vi "Log.vi"(10 "Log Packet":T1, 11 "String Log Sink in":refnum<class "String Log Sink.lvclass">) -> (0 "error out":errorcluster, 3 "String Log Sink out":refnum<class "String Log Sink.lvclass">)   [LabVIEW 2019, in "String Log Sink.lvclass"]
uses:
  <vilib>/gpm_packages/@cs/event-logger/Source/String Log Sink/String Log Sink.lvclass
  <vilib>/gpm_packages/@cs/event-logger/Source/Composed Log/Types/Log Packet.ctl
  <vilib>/gpm_packages/@cs/event-logger/Source/Composed Log/Types/Log Level.ctl
  <vilib>/gpm_packages/@cs/event-logger/Source/String Log Sink/String Log Sink.lvclass/String Log Sink.ctl
  <vilib>/gpm_packages/@cs/event-logger/Source/IStringFormat/IStringFormat.lvclass
  <vilib>/gpm_packages/@cs/event-logger/Source/Composed Log/Composed Log.lvlib
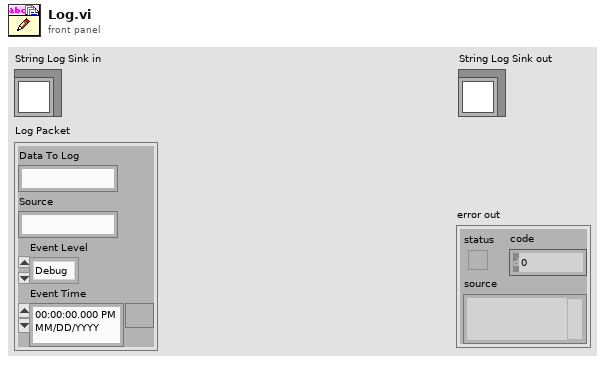
[diagram p1: front panel]
types:
  T1 = typedef "Composed Log.lvlib/Log Packet.ctl" = cluster{"Data To Log":string, "Source":string, "Event Level":T2, "Event Time":timestamp}
  T2 = typedef "Composed Log.lvlib/Log Level.ctl" = enum16{"Debug", "Info", "Warning", "Error", "Critical"}
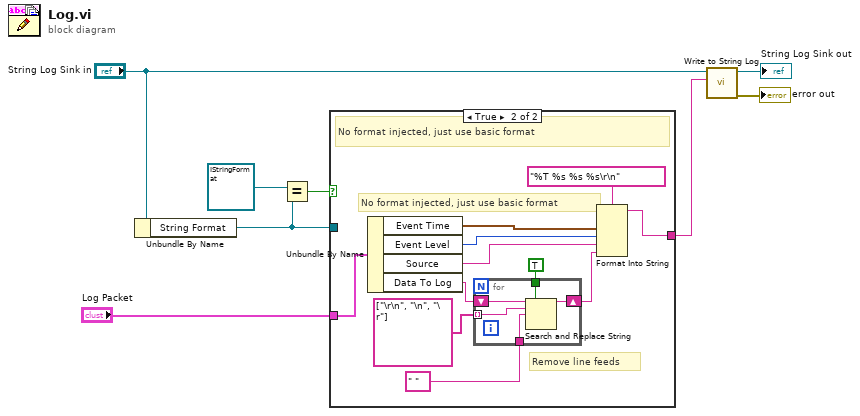
[diagram p0: block diagram]
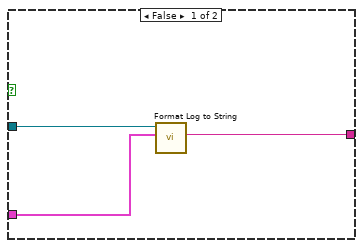
[diagram p2: hidden frame]
diagram:
  n1 = Unbundle By Name("String Log Sink in") -> ("String Format"=w6:refnum<class "IStringFormat.lvclass">)
  n2 = Equal?(x=refnum<class "IStringFormat.lvclass"> refnum ("y"), y=w6) -> (x = y?=w7:bool)
  n3 = case shown="True" w7 {
    tunnel: w6 -> [w11 _]
    tunnel: "Log Packet" -> [w10 w13]
    tunnel: [w9 w12] -> w2
    frame False {
      n4 = call-dynamic "Format Log to String.vi"("Log Packet"=w10, "IStringFormat in"=w11) -> ("Log Entry"=w9:string)  [unwired: 8 in, 1 out]
    }
    frame True {
      # "Remove line feeds"
      # "No format injected, just use basic format"
      # "No format injected, just use basic format"
      n5 = Unbundle By Name(w13) -> ("Event Time"=w22:timestamp, "Event Level"=w20:T2, "Source"=w19:string, "Data To Log"=w18:string)
      n6 = for {
        shift-right: [w26] -> w17
        shift-left: w18 -> [w27]
        tunnel: TRUE ("replace all? (F)") -> [w25]
        tunnel: string[] ["\r\n", "\n", "\r"] ("search string") -> [w24] mode=indexing
        tunnel: " " ("replace string (\"\")") -> [w23]
        n7 = Search and Replace String(replace all?=w25, input string=w27, search string=w24, replace string=w23) -> (result string=w26:string)  [unwired: 4 in, 3 out]
      }
      n8 = Format Into String(format string="%T %s %s %s\r\n", w22, w20, w19, w17) -> (resulting string=w12:string)  [unwired: 2 in, 1 out]
    }
  }
  n9 = call-dynamic "Write to String Log.vi"("String to Log"=w2, "String Log Sink in"="String Log Sink in") -> ("error out"=→"error out":errorcluster, "String Log Sink out"=→"String Log Sink out":refnum<class "String Log Sink.lvclass">)  [unwired: 8 in]
